vi "TBM.SetDimmer.vi"(5 "Dim Transparency":u8, 7 "DimRegion":enum16{"VI", "Control", "Screen"}(ring), 8 "error in (no error)":errorcluster, 9 "Ctrl Screen Bounds":T1, 10 "FP Screen Bounds":T1) -> (0 "error out":errorcluster, 3 "Dimmer VI out":refnum<vi>)   [LabVIEW 2013, in "ToolbarMenu.lvlib"]
uses:
  ToolbarMenu.lvlib
  <vilib>/Utility/miscctls.llb/LVRectTypeDef.ctl
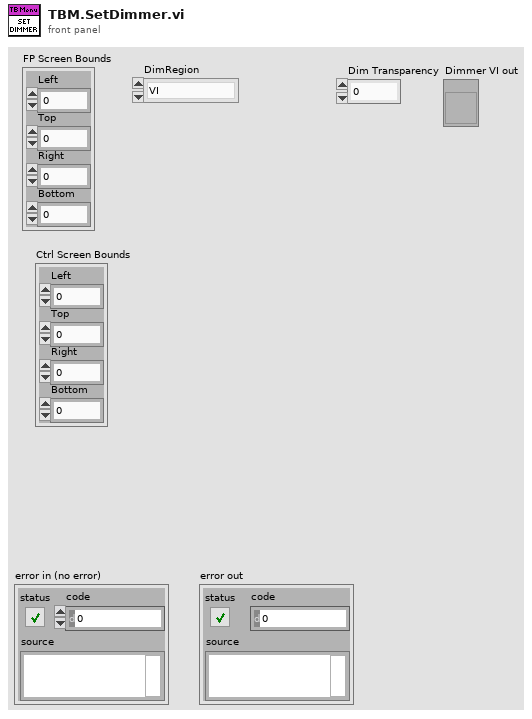
[diagram p1: front panel]
types:
  T1 = typedef "LVRectTypeDef.ctl" = cluster{"Left":i16, "Top":i16, "Right":i16, "Bottom":i16}
  T2 = enum32{"Invalid", "Standard", "Closed", "Hidden", "Minimized", "Maximized"}
  T3 = cluster{"Left":i16, "Top":i16, "Right":i16, "Bottom":i16}
  T4 = typedef "LVAllMonitorsDisplayTypeDef.ctl" = cluster{"Bounds":cluster{"Left":i16, "Top":i16, "Right":i16, "Bottom":i16}, "Depth":i16}[]
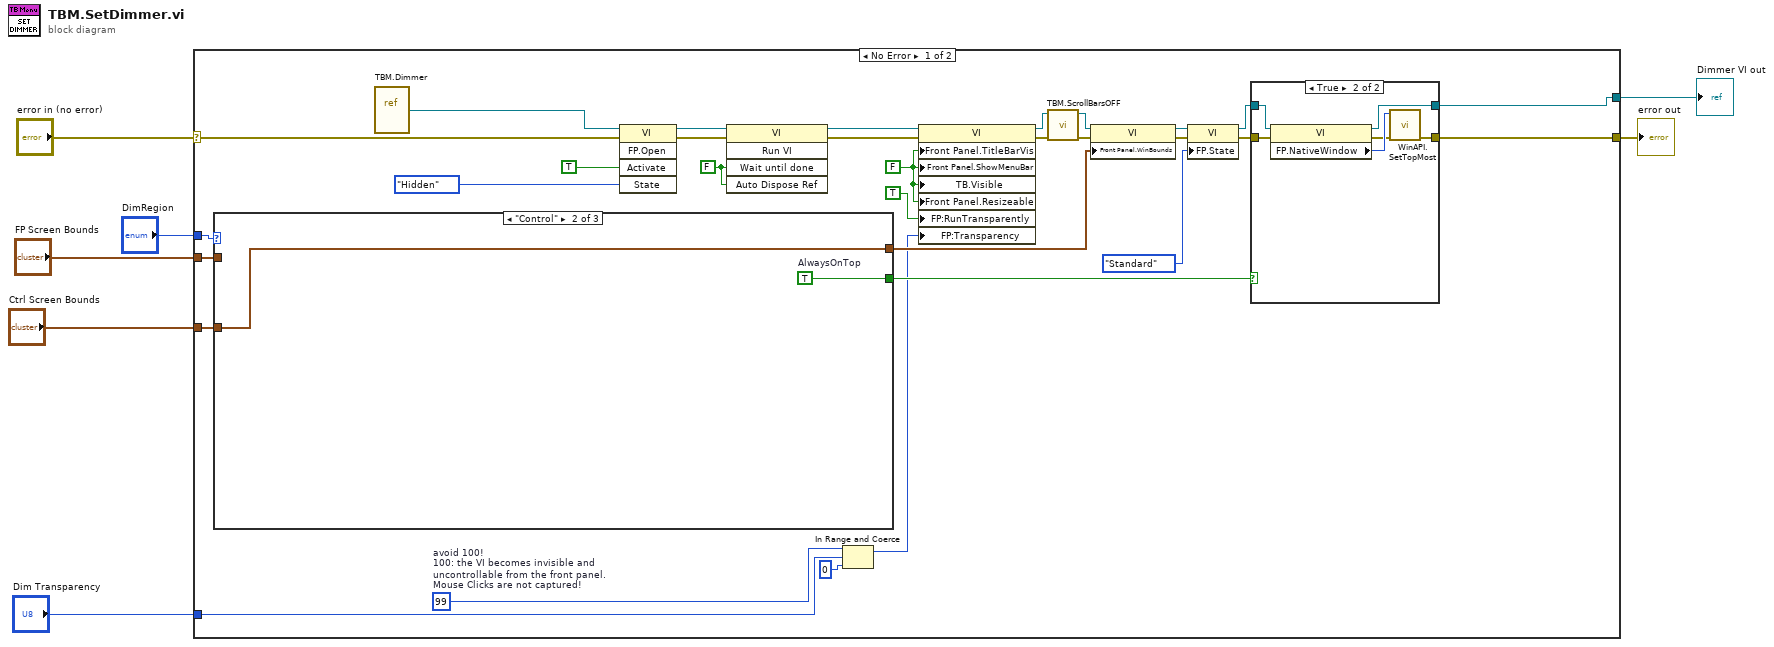
[diagram p0: block diagram]
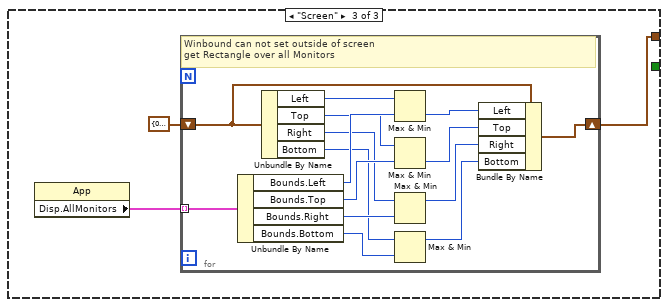
[diagram p4: hidden frame]
diagram:
  n1 = case shown="No Error" "error in (no error)" {
    selector: "error in (no error)" -> [w24 w68]
    tunnel: [w8 _] -> w7
    tunnel: [w9 w68] -> w6
    tunnel: "DimRegion" -> [w23 _]
    tunnel: "FP Screen Bounds" -> [w22 _]
    tunnel: "Ctrl Screen Bounds" -> [w21 _]
    tunnel: "Dim Transparency" -> [w20 _]
    frame No Error {
      w29 = FALSE ("Front Panel Window:Run VI Transparently")
      w36 = u8 99  # avoid 100! 100: the VI becomes invisible and uncontrollable from the front panel. Mouse Clicks are not captured!
      w34 = FALSE ("Front Panel Window:Run VI Transparently")
      n2 = case shown="\"Control\"" w23 {
        tunnel: w22 -> [w47 _ _]
        tunnel: [w47 w49 w51] -> w30
        tunnel: w21 -> [_ w49 _]
        tunnel: [_ w48 _] -> w19
        frame "VI" {
        }
        frame "Control" {
          w48 = TRUE  # AlwaysOnTop
        }
        frame "Screen" {
          n3 = property class="App"() -> ("Disp.AllMonitors"=w52:T4)  [unwired: 2 in, 2 out]
          n4 = for {
            tunnel: w52 -> [w67] mode=indexing
            shift-right: [w65] -> w51
            shift-left: T3 {"Left"=0, "Top"=0, "Right"=0, "Bottom"=0} ("Bounds") -> [w66]
            # "Winbound can not set outside of screen\nget Rectangle over all Monitors"
            n5 = Unbundle By Name(w67) -> ("Bounds.Left"=w63:i16, "Bounds.Top"=w59:i16, "Bounds.Right"=w55:i16, "Bounds.Bottom"=w53:i16)
            n6 = Unbundle By Name(w66) -> ("Left"=w64:i16, "Top"=w60:i16, "Right"=w56:i16, "Bottom"=w54:i16)
            n7 = Max & Min(x=w64, y=w63) -> (min(x,y)=w62:i16)  [unwired: 1 out]
            n8 = Max & Min(x=w60, y=w59) -> (min(x,y)=w61:i16)  [unwired: 1 out]
            n9 = Max & Min(x=w56, y=w55) -> (max(x,y)=w58:i16)  [unwired: 1 out]
            n10 = Max & Min(x=w54, y=w53) -> (max(x,y)=w57:i16)  [unwired: 1 out]
            n11 = Bundle By Name(cluster=w66, "Left"=w62, "Top"=w61, "Right"=w58, "Bottom"=w57) -> (w65:T3)
          }
        }
      }
      n12 = vi-ref "TBM.Dimmer.vi"() -> (w35:refnum<vi>)
      n13 = invoke class="VI" method="FP.Open"(reference=w35, error in=w24, "Activate"=TRUE ("Activate?"), "State"=T2."Hidden") -> (reference out=w33:refnum<vi>, error out=w38:errorcluster)  [unwired: 1 in, 3 out]
      n14 = invoke class="VI" method="Run VI"(reference=w33, error in=w38, "Wait until done"=w34, "Auto Dispose Ref"=w34) -> (reference out=w28:refnum<vi>, error out=w16:errorcluster)  [unwired: 1 in, 3 out]
      n15 = In Range and Coerce(upper limit=w36, x=w20, lower limit=u8 0 ("upper limit")) -> (coerced(x)=w10:u8)  [unwired: 1 out]
      n16 = property class="VI"(reference=w28, error in=w16, "Front Panel.TitleBarVis"=w29, "Front Panel.ShowMenuBar"=w29, "TB.Visible"=w29, "Front Panel.Resizeable"=w29, "FP:RunTransparently"=TRUE ("Front Panel Window:Run VI Transparently"), "FP:Transparency"=w10) -> (reference out=w15:refnum<vi>, error out=w13:errorcluster)
      n17 = call "TBM.ScrollBarsOFF.vi"("error in (no error)"=w13, "VI in"=w15) -> ("error out"=w12:errorcluster, "VI out"=w14:refnum<vi>)  [unwired: 8 in]
      n18 = property class="VI"(reference=w14, error in=w12, "Front Panel.WinBounds"=w30) -> (reference out=w27:refnum<vi>, error out=w26:errorcluster)
      n19 = property class="VI"(reference=w27, error in=w26, "FP.State"=T2."Standard" ("Front Panel Window:State")) -> (reference out=w18:refnum<vi>, error out=w17:errorcluster)
      n20 = case shown="True" w19 {
        tunnel: w18 -> [w40 w46]
        tunnel: [w40 w43] -> w8
        tunnel: w17 -> [w39 w42]
        tunnel: [w39 w41] -> w9
        frame False {
        }
        frame True {
          n21 = property class="VI"(reference=w46, error in=w42) -> (reference out=w43:refnum<vi>, error out=w44:errorcluster, "FP.NativeWindow"=w45:u64)
          n22 = call "WinAPI.SetTopMost.vi"("error in (no error)"=w44, "hWnd"=w45) -> ("error out"=w41:errorcluster)  [unwired: 9 in]
        }
      }
    }
    frame Error {
    }
  }
  "error out" <- w6
  "Dimmer VI out" <- w7
